vi "Potentiometer Control-Lift.vi"(11 "Enum":T1) -> (3 "Normalized Value":dbl)   [LabVIEW 2014]
uses:
  TypeDefs/SRE Enum.ctl
  <vilib>/Rock Robotics/SystemInterfaces/AI/FPGA_AIChannel.ctl
  <vilib>/Rock Robotics/WPI/Power/WPI_Power Get 5Volt Rail Voltage and Current.vi
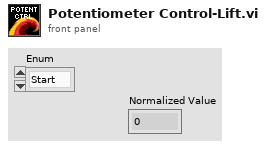
[diagram p1: front panel]
types:
  T1 = typedef "SRE Enum.ctl" = enum16{"Start", "Run", "End"}
  T2 = typedef "FPGA_AIChannel.ctl" = enum8{"AI 0", "AI 1", "AI 2", "AI 3", "AI MXP 0", "AI MXP 1", "AI MXP 2", "AI MXP 3", "Invalid"}
  T3 = typedef "WPI_AnalogChannelDevRef.ctl" = cluster{"DevStatus":errorcluster, "Controller":T4, "Analog Channel":T2}
  T4 = typedef "FPGA_TypedefAnalogModule.ctl" = enum16{"Controller 1"}
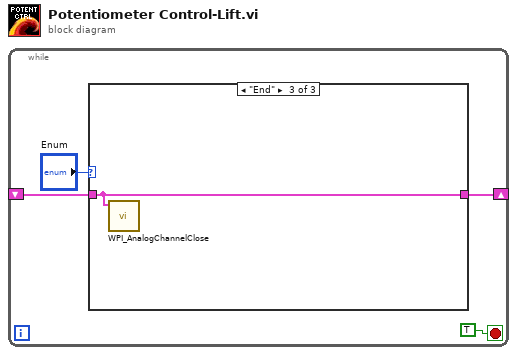
[diagram p0: block diagram]
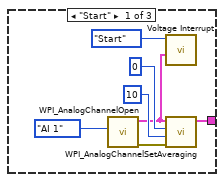
[diagram p2: hidden frame]
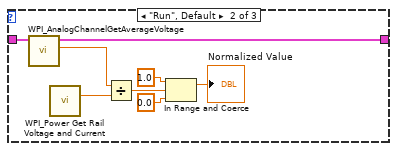
[diagram p3: hidden frame]
diagram:
  n1 = while {
    shift-right: [w2] -> _
    shift-left: _ -> [w1]
    stop <- TRUE stop-if-true
    n2 = case shown="\"End\"" "Enum" {
      tunnel: [w5 w12 w20] -> w2
      tunnel: w1 -> [_ w19 w20]
      frame "Start" {
        n3 = call <vilib>:"WPI_AnalogChannelOpen.vi"("Analog Channel"=FPGA_AIChannel."AI 1") -> ("error out"=w10:errorcluster, "AIDeviceRef"=w7:T3)  [unwired: 9 in]
        n4 = call "Voltage Interrupt.vi"("AnalogTriggerSource"=w7, "Enum"=SRE_Enum."Start") -> ()  [unwired: 10 in]
        n5 = call <vilib>:"WPI_AnalogChannelSetAveraging.vi"("error in (no error)"=w10, "OversampleBits"=u8 10, "AverageBits"=u8 0, "AIDeviceRef"=w7) -> ("AIDeviceRef"=w5:T3)  [unwired: 6 in, 1 out]
      }
      frame "Run", Default {
        n6 = call <vilib>:"WPI_AnalogChannelGetAverageVoltage.vi"("AIDeviceRef"=w19) -> ("Voltage"=w18:dbl, "AIDeviceRef"=w12:T3)  [unwired: 8 in, 1 out]
        n7 = call-poly <vilib>:"WPI_Power Get Rail Voltage and Current.vi"() -> ("5 volt rail voltage (V)"=w17:dbl)  [unwired: 13 in, 2 out]
        n8 = Divide(x=w18, y=w17) -> (x/y=w14:dbl)
        n9 = In Range and Coerce(upper limit=1.0, x=w14, lower limit=0.0) -> (coerced(x)=→"Normalized Value":dbl)  [unwired: 1 out]
      }
      frame "End" {
        n10 = call <vilib>:"WPI_AnalogChannelClose.vi"("AIDeviceRef"=w20) -> ()  [unwired: 10 in, 1 out]
      }
    }
  }
